vi "SiPM_Data_Analysis.vi"() -> ()   [LabVIEW 2019]
uses:
  <vilib>/Utility/error.llb/DialogType.ctl
  SiPM_Tests_Global_Var.vi
  Data_Analysis_subvis/ESA_Data_Analysis_Global_VIs.vi
  <vilib>/Analysis/NI_AALPro.lvlib
panel:
  out "property names":string[](array[string])
  out "property values":variant[](array[variant])
  out "data":waveform(dbl)[](array[waveform])
  out "Indicator":bool
  in  "Close Session":bool
  in  "Spectrum Calculation":bool=TRUE
  in  "Waveform Nb":u16
  in  "NbSamples":i64=100000 caption="Nb of Samples to Analyze" format="%.0p"
  in  "Refresh":bool
  in  "Load file to display":bool
  in  "Detailed":bool
  in  "Listbox":i32[](listbox) caption="Protn-Neutron_Board_v1.tdms"
  in  "Y-Scale":bool
  out "Nb of Selected Events":dbl step=0.001 format="%#_6p"
  out "Total Nb of Recorded Events":dbl step=0.001 format="%#_6p"
  in  "CH4 Trigger Logic":T1(ring)
  in  "CH4 Trigger Thr":dbl=0.003 caption="CH4 Trigger Thr (V)" step=0.001 format="%#_6p"
  in  "CH3 Trigger Logic":T1(ring)
  in  "CH3 Trigger":dbl=0.003 caption="CH3 Trigger Thr (V)" step=0.001 format="%#_6p"
  in  "CH2 Trigger Logic":T1(ring)
  in  "CH2 Trigger Thr":dbl=0.003 caption="CH2 Trigger Thr (V)" step=0.001 format="%#_6p"
  in  "AutoScale 3":bool
  in  "Update Energy":bool
  out "Energy_Spectr":T2(graph) caption="Spectrum"
  in  "Filter \nON?":bool
  in  "Threshold 2":dbl caption="Max_Value (V)" step=0.001 format="%#_6p"
  in  "Threshold":dbl caption="Energy Threshold (V)" step=0.001 format="%#_6p"
  out "SiPM Waveform":waveform(dbl)[](graph)
  out "Table":string[][](table)
  in  "Bin Min (V)":dbl=-0.0042 step=0.001 format="%#_6p"
  in  "Bin Max (V)":dbl=0.03005 step=0.001 format="%#_6p"
  out "Nb of Channels in Group":i32
  out "group names":string[](array[string])
  out "tdms file out":refnum<k34>
  in  "File contents":string[](tree)
  # "NCSR  DEMOKRITOS\nInstitute of Nuclear and Particle Physics\nDetectors Instrumentation Laboratory"
  # "SiPM Data Analysis"
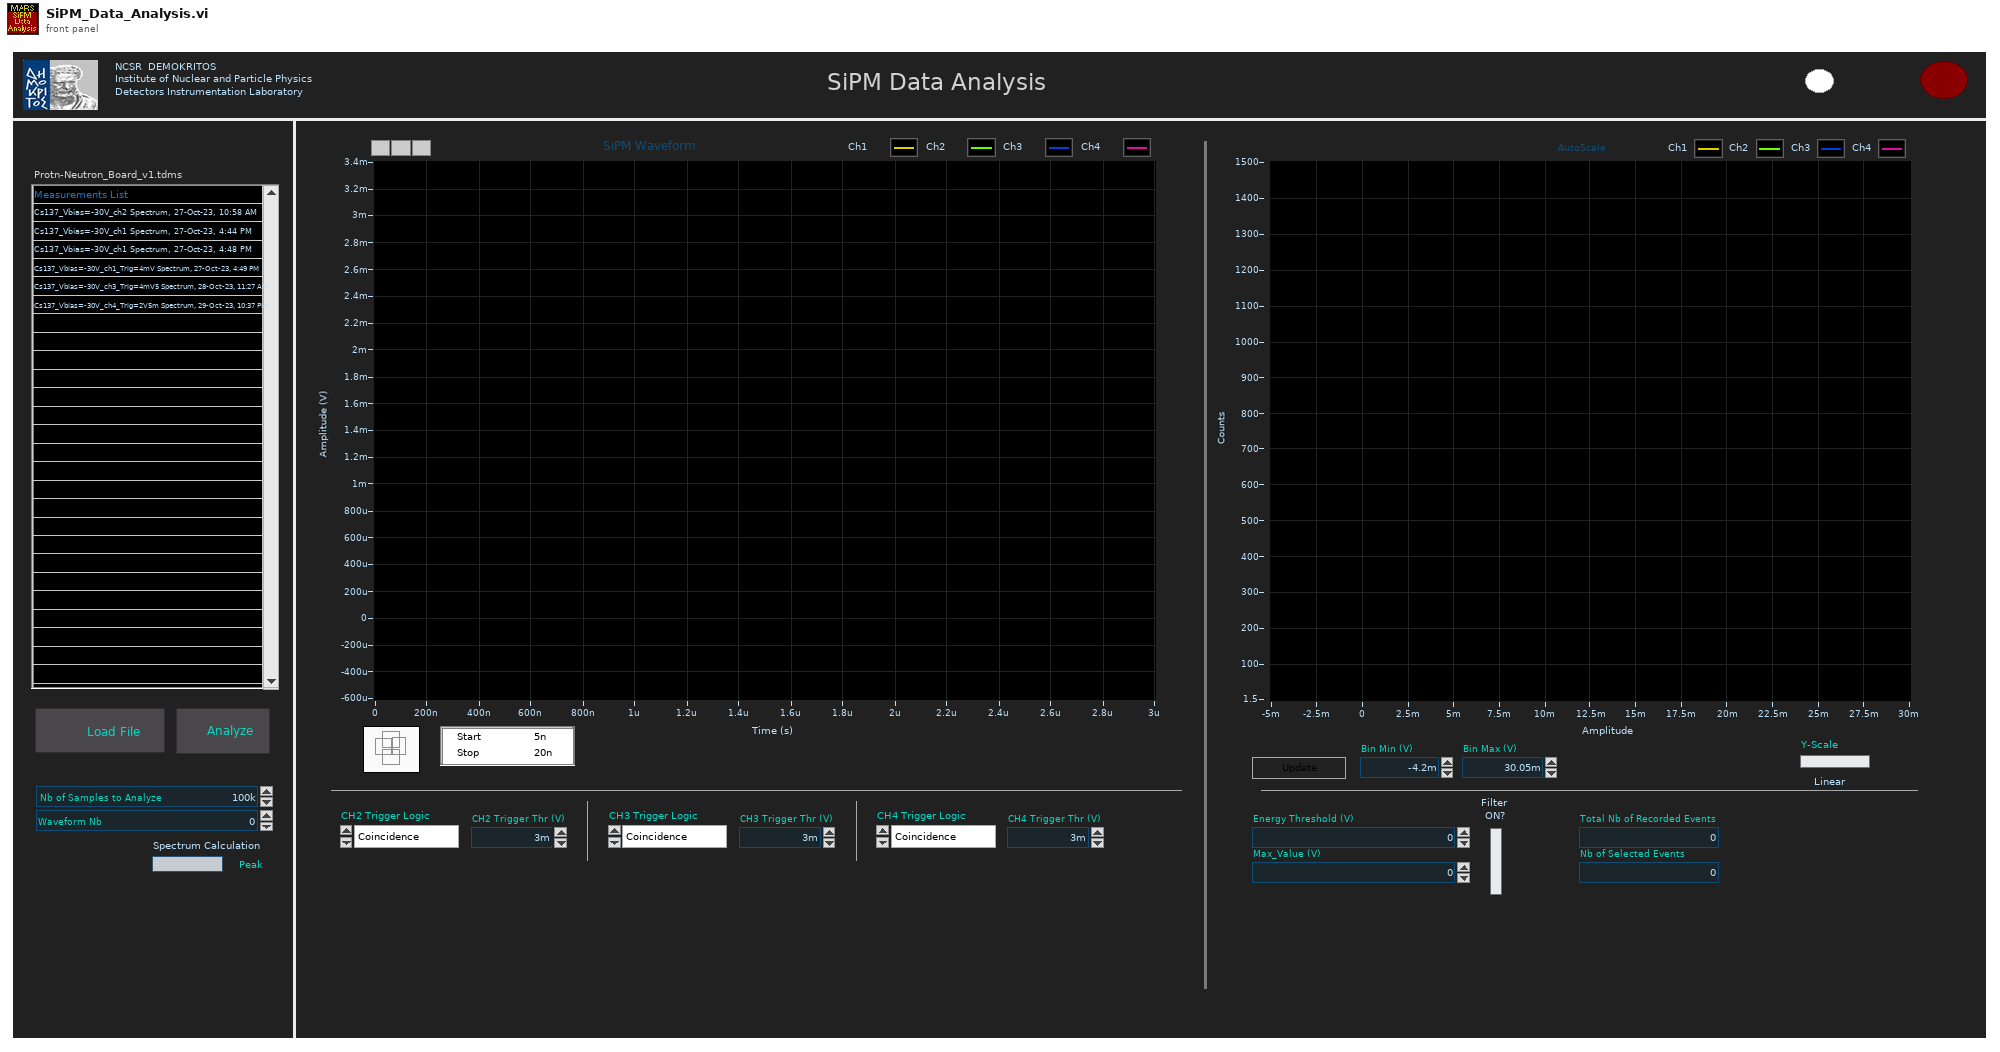
[diagram p1: front panel]
types:
  T1 = enum16{"Coincidence", "Anti-Coincidence", "Don't Care"}
  T2 = cluster{"X Values":dbl[], "Histogram: h(x)":i32[]}[]
  T3 = typedef "DialogType.ctl" = u16
  T4 = enum16{"open", "open or create", "create or replace", "create", "open (read-only)"}
  T5 = cluster{"X Values":dbl[], "Histogram: h(x)":i32[]}
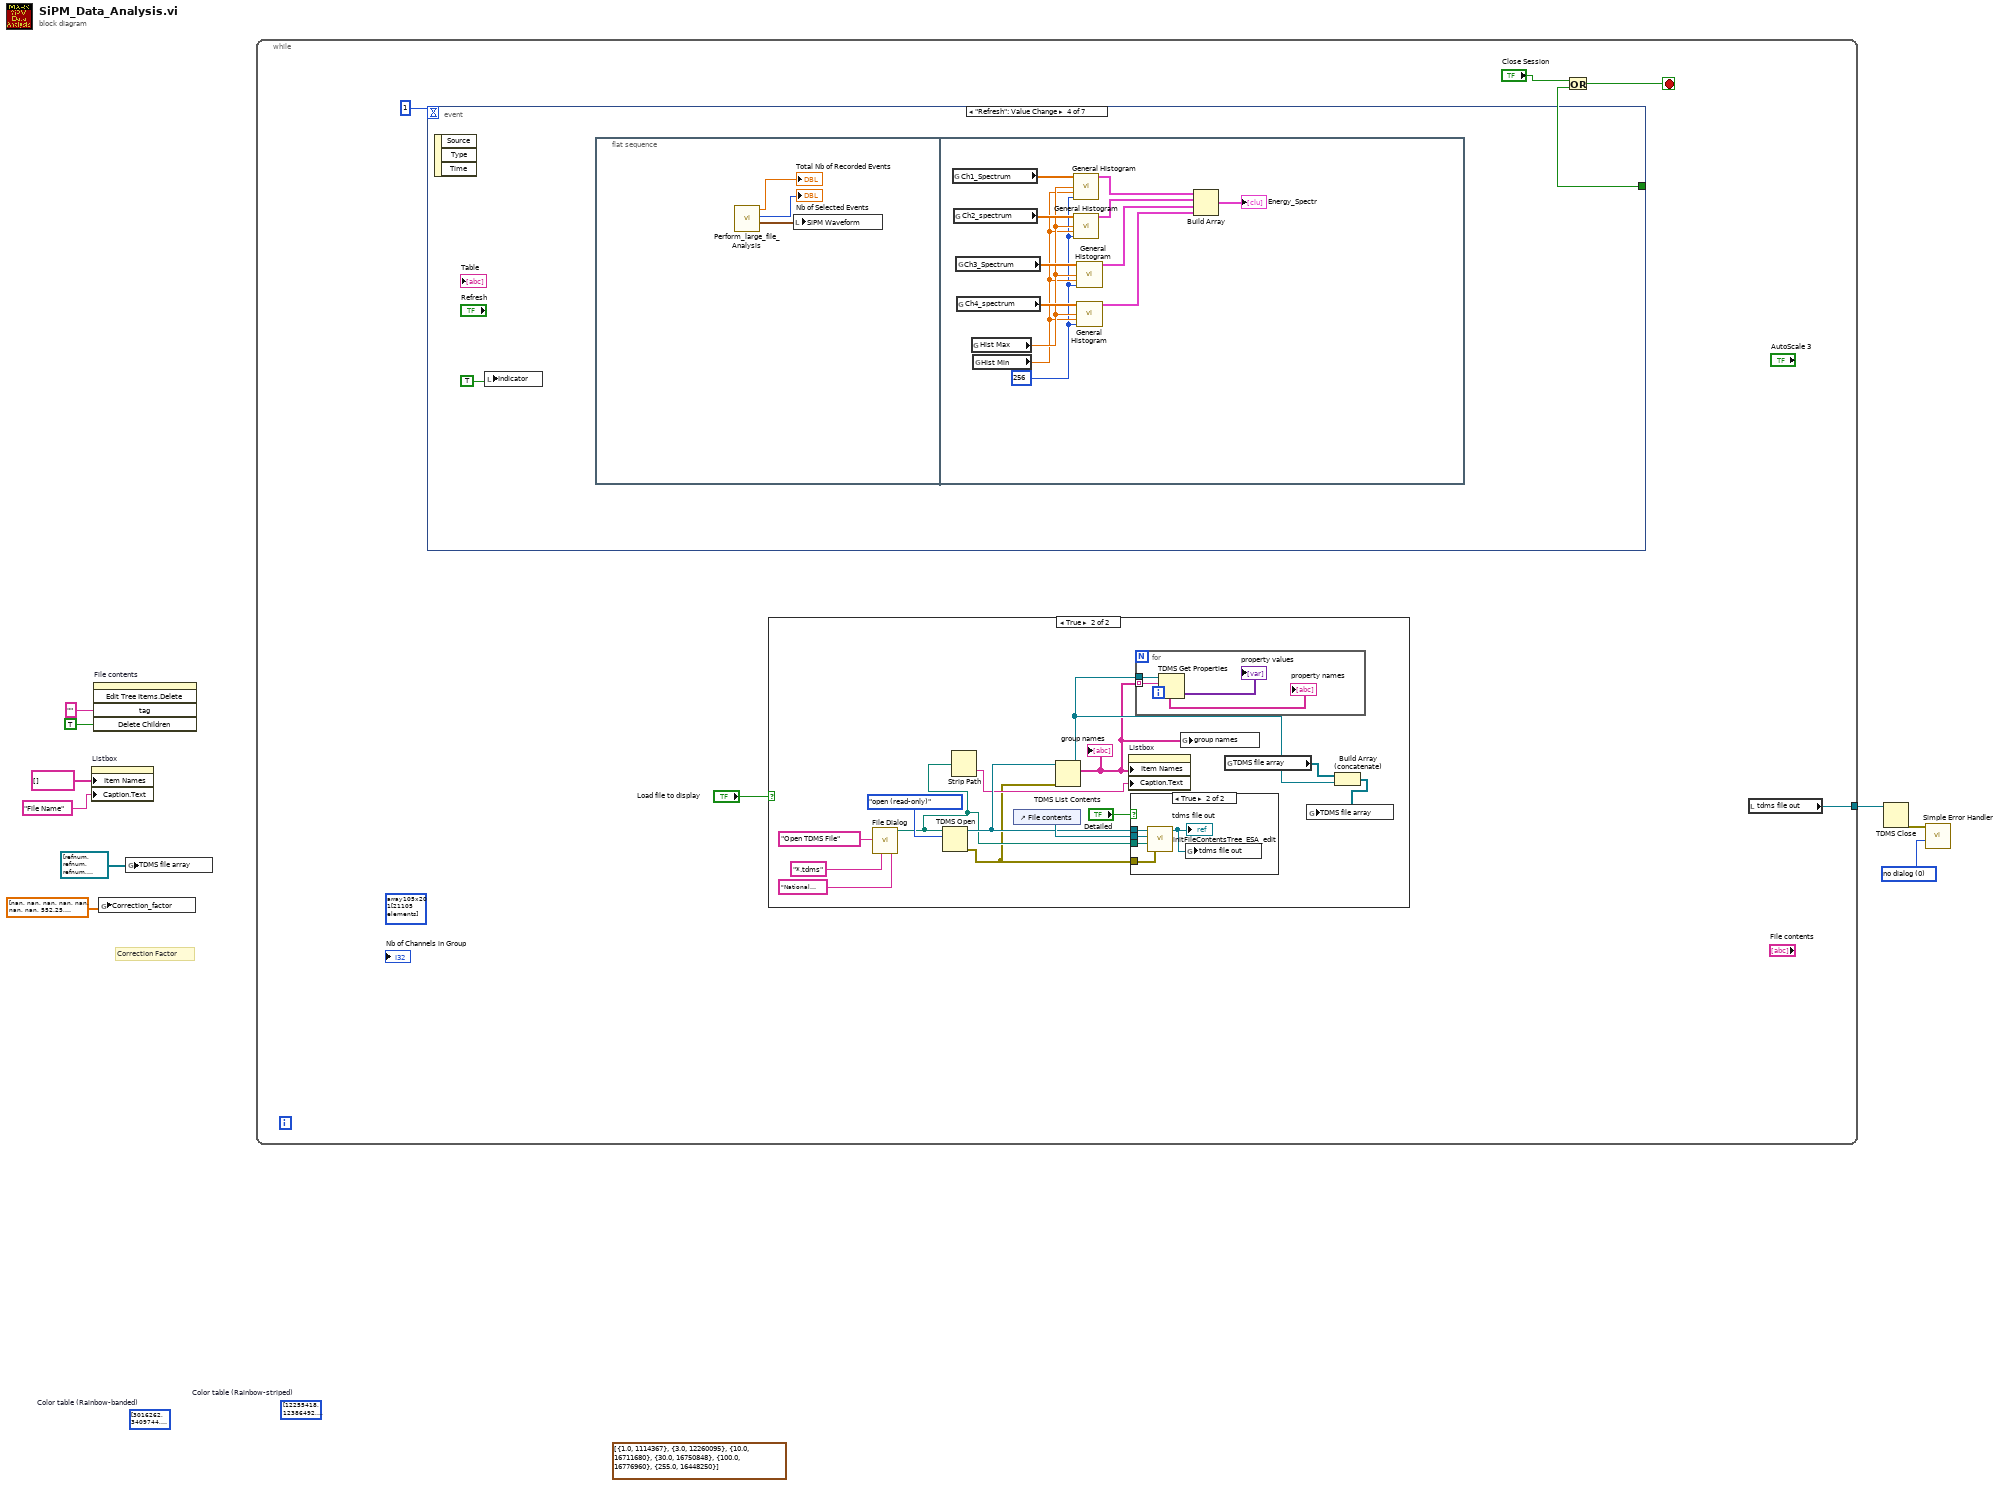
[diagram p0: block diagram]
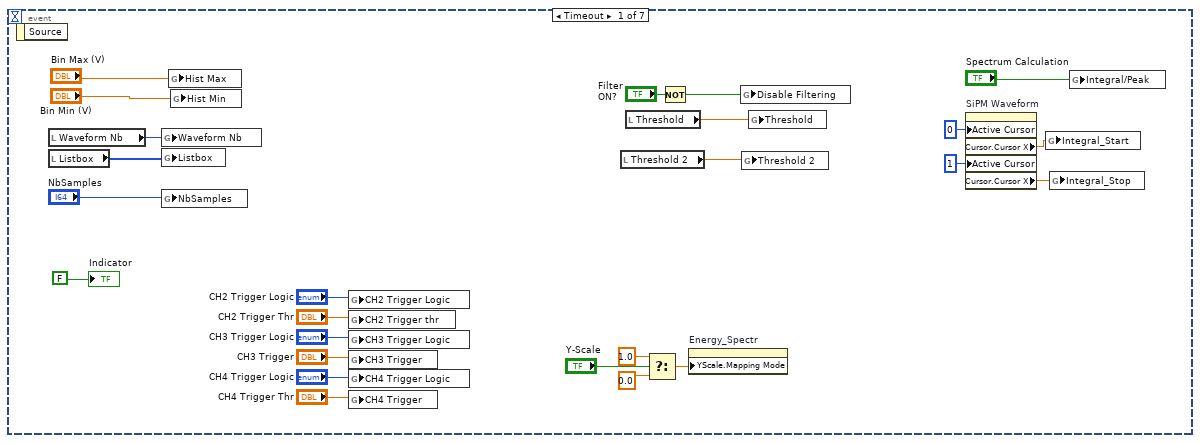
[diagram p2: hidden frame]
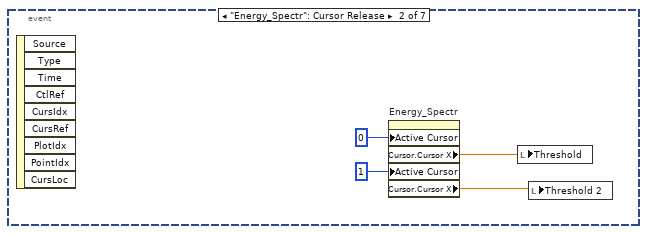
[diagram p3: hidden frame]
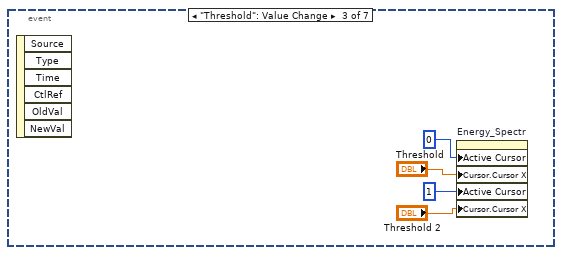
[diagram p4: hidden frame]
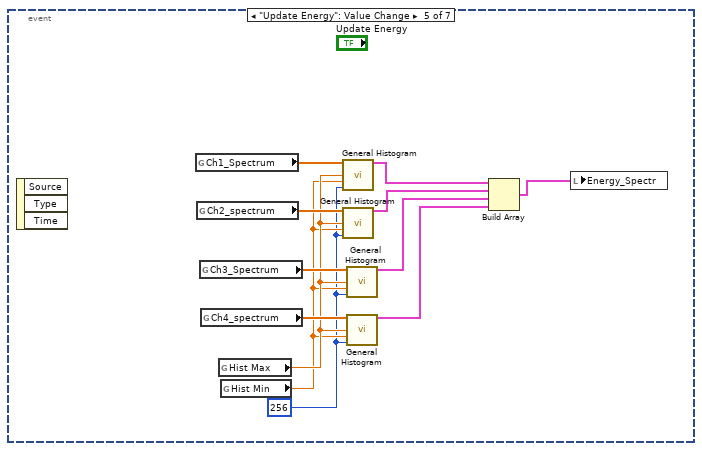
[diagram p5: hidden frame]
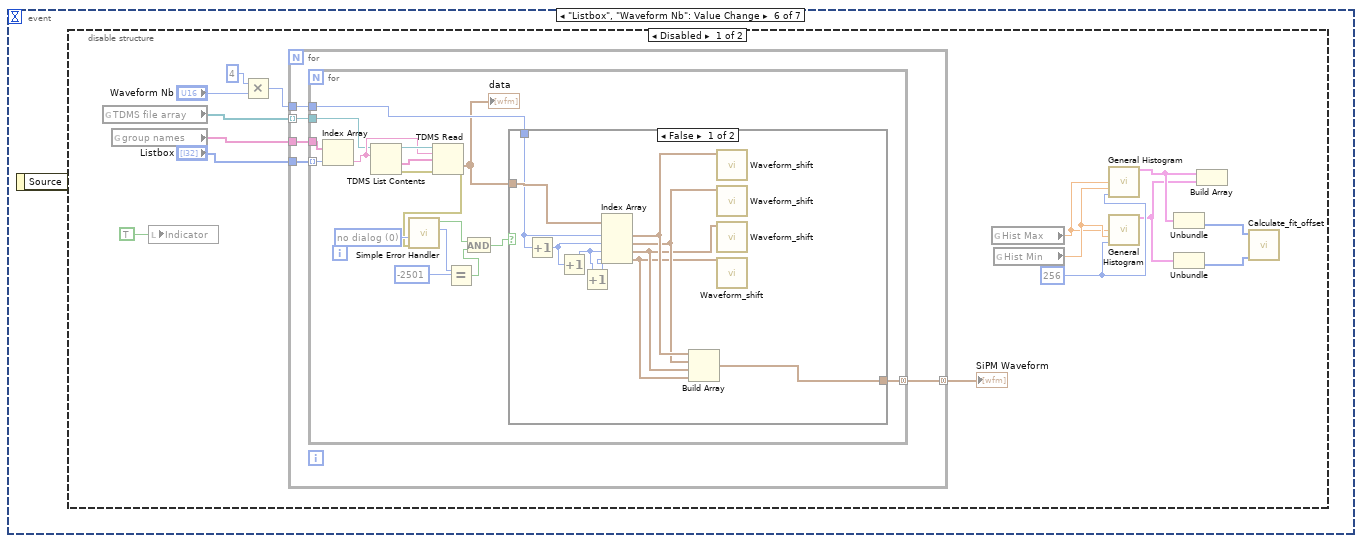
[diagram p6: hidden frame]
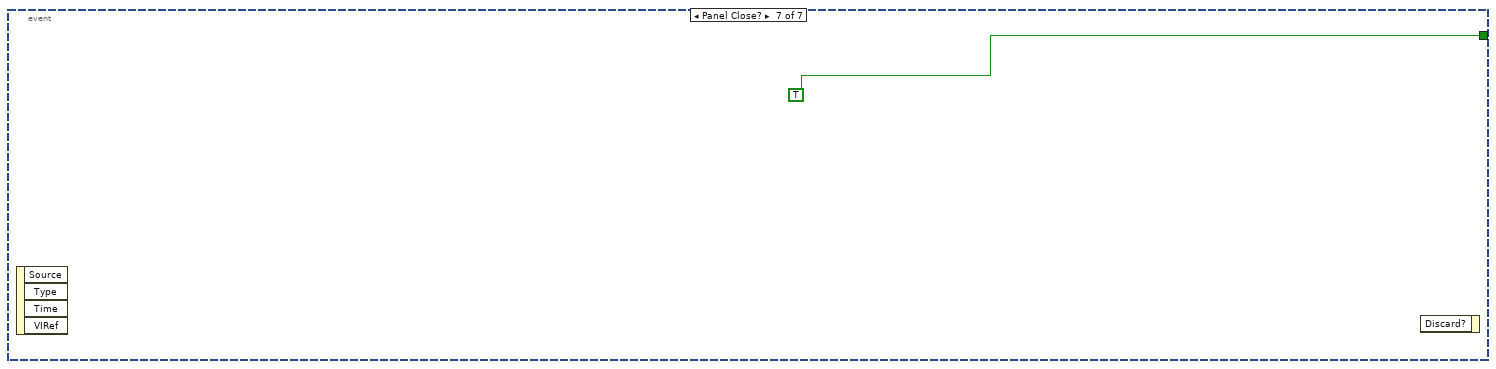
[diagram p9: hidden frame]
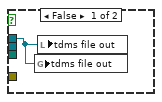
[diagram p11: hidden frame]
diagram:
  w2 = T3 0 items=["no dialog", "OK message", "continue or stop message", "OK message + warnings", "continue/stop + warnings"] ("type of dialog (OK msg:1)")
  (unwired) cluster{dbl, u32}[] [{1.0, 1114367}, {3.0, 12260095}, {10.0, 16711680}, {30.0, 16750848}, {100.0, 16776960}, {255.0, 16448250}] ("Z Scale.Marker Values[]")
  (unwired) u32[] [12255418, 12386492, 12517567, 12320960, 12189888, 12058817, 11927746, 11731139, 11600067, 9175197, 9044125, 11141318, 11010246, 10813639, 10682568, 10551497, 10354890, 10223818, 10092747, 7930019, 7798948, 9633997, 9502926, 9306319, 9175248, 9044176, 8847569, 8716498, 8585427, 6750377, 6619306, 8126677, 7995606, 7798999, 7667927, 7536856, 7340249, 7209178, 7078106, 5505199, 5374128, 6619357, 6488285, 6291678, 6160607, 6029536, 5832929, 5701857, 5570786, 4325557, 4194486, 5112036, 4980965, 4784358, 4653287, 4522215, 4325608, 4194537, 4063466, 3080380, 3014844, 3604716, 3408109, 3277038, 3277038, 3145966, 3014895, 2818288, 2687217, 2556145, 1900738, 1769666, 2097396, 1900789, 1769717, 1638646, 1507575, 1310968, 1179896, 1048825, 721096, 590024, 590075, 393468, 262397, 131326, 255, 1791, 3327, 4863, 5068, 6348, 9471, 11007, 12543, 14079, 15615, 17151, 18687, 20223, 17612, 18636, 25087, 26623, 28159, 29695, 31231, 32767, 34303, 35839, 29900, 31180, 40447, 41983, 43775, 45311, 46847, 48383, 49919, 51455, 42444, 43724, 56063, 57599, 59135, 60671, 62207, 63743, 65535, 65528, 52418, 52413, 65510, 65504, 65498, 65492, 65486, 65480, 65474, 65468, 52369, 52364, 65449, 65443, 65437, 65431, 65425, 65419, 65413, 65407, 52321, 52316, 65389, 65383, 65377, 65371, 65364, 65358, 65352, 65346, 52272, 52267, 65328, 65322, 65316, 65310, 65304, 65298, 65292, 65286, 52224, 314368, 851712, 1244928, 1638144, 2031360, 2424576, 2817792, 3211008, 3604224, 3197952, 3525632, 4783872, 5177088, 5635840, 6029056, 6422272, 6815488, 7208704, 7601920, 6409216, 6736896, 6736896, 8781568, 9174784, 9568000, 9961216, 10354432, 10747648, 11206400, 11599616, 9554944, 9882624, 12779264, 13172480, 13565696, 13958912, 14352128, 14745344, 15138560, 15531776, 12766208, 13093888, 16776960, 16775170, 16773637, 16771847, 16770314, 16768780, 16766991, 16765457, 13411088, 13409810, 16760601, 16758812, 16757278, 16755745, 16753955, 16752422, 16750888, 16749099, 13398052, 13396774, 16744243, 16742704, 16741166, 16739884, 16738345, 16736807, 16735269, 16733730, 13385753, 13384728, 16729371, 16727833, 16726295, 16725012, 16723474, 16721936, 16720397, 16718859, 13373959, 13372677, 16714500, 16712962, 16711680]  # Color table (Rainbow-striped)
  (unwired) u32[] [3016262, 3409744, 4000097, 4721526, 5508493, 6229924, 6820281, 7214025, 7345364, 7279831, 6886611, 6362057, 5640632, 4788132, 4001165, 3214197, 2492769, 2033488, 1640006, 1508930, 1508934, 1640272, 1902945, 2165622, 2428301, 2690980, 2822585, 2888649, 2757844, 2626775, 2299091, 1971145, 1642936, 1249188, 920973, 724086, 592737, 461392, 395846, 396098, 396358, 462928, 595297, 727925, 861069, 994212, 1127608, 1260745, 1328083, 1329111, 1329876, 1264073, 1132217, 999844, 866957, 734070, 600929, 468304, 401734, 401730, 402502, 469584, 603489, 737909, 737909, 872845, 1008036, 1143224, 1277641, 1345747, 1347287, 1347796, 1281225, 1147833, 1013668, 878989, 743798, 609121, 475216, 407878, 407362, 408390, 476496, 611681, 747893, 884877, 1022116, 1158840, 1294793, 1363667, 1365719, 1365202, 1296836, 1161649, 1025178, 888194, 751211, 614742, 479302, 411196, 410168, 411193, 479297, 614732, 750939, 888171, 1025145, 1161350, 1296782, 1364883, 1365906, 1365132, 1296769, 1161588, 1025124, 888147, 751172, 614710, 479276, 411173, 410146, 411170, 479270, 614700, 750900, 888124, 1025091, 1161289, 1296716, 1364813, 1365834, 1365062, 1296703, 1161527, 1025070, 888101, 751133, 614678, 479249, 411149, 410124, 411147, 479244, 614668, 750861, 888078, 1156111, 1488913, 1820947, 2151188, 2414356, 2610196, 2738451, 2668817, 2597903, 2329869, 2061835, 1794313, 1593351, 1459718, 1458694, 1590790, 1921031, 2449673, 3110155, 3902733, 4695055, 5486609, 6211859, 6738708, 7132948, 7197716, 7063827, 6666513, 6136847, 5410061, 4617739, 3957001, 3362823, 2967046, 2900486, 3098118, 3690503, 4546825, 5666059, 6917389, 8233999, 9484305, 10537235, 11326228, 11786004, 11785236, 11785236, 11454739, 10729745, 9675791, 8424717, 7173643, 6054153, 5066759, 4474374, 4342278, 4605190, 5262855, 6380553, 7695883, 9273613, 10785807, 12100625, 13217555, 13874452, 14136340, 13938196, 13214227, 12161553, 10780431, 9267725, 7755531, 6374921, 5257479, 4599814, 4336646, 4599302, 5255943, 6372361, 7685899, 9261837, 10771983, 12085009, 13200659, 13856532, 14118164, 13920276, 13197075, 12145937, 10766351, 9255949, 7745547, 6366729, 5250567, 4593926, 4331014, 4593158, 5249287, 6364169, 7675915, 9249805, 10758159, 12069393, 13183507, 13838612, 14099988, 13902356, 13180179, 12130065, 10752527]  # Color table (Rainbow-banded)
  # "Correction Factor"
  n1 = property on="Listbox" class="LstBox (strict)"("Item Names"=string[] [], "Caption.Text"="File Name") -> ()  [unwired: 2 in, 2 out]
  n2 = invoke on="File contents" class="Tree (strict)" method="Edit Tree Items.Delete"("tag"="" ("Tag"), "Delete Children"=TRUE ("Delete Children?")) -> ()  [unwired: 3 in, 5 out]
  n3 = global write "SiPM_Tests_Global_Var.vi" "Correction_factor"(dbl[] [nan, nan, nan, nan, nan, nan, nan, 552.25, 547.2727272727273, 556.8888888888889, 571.6521739130435, 581.5526315789474, 593.6590909090909, 606.7333333333333, 610.4848484848485, 619.9565217391304, 624.8125, 628.375, 631.8064516129032, 637.0434782608696, 640.92, 643.5, 643.92, 647.7619047619048, 650.1923076923077, 651.5714285714286, 652.375, 654.9130434782609, 656.35, 658.4117647058823, 658.5909090909091, 660.0952380952381, 662.3157894736842, 661.5, 663.4166666666666, 665.8888888888889, 666.0, 666.0, 667.8421052631579, 668.2727272727273, 669.7, 671.4166666666666, 671.2631578947369, 672.2272727272727, 672.0588235294117, 674.0952380952381, 673.0, 674.0526315789474, 675.6111111111111, 677.1578947368421, 677.9411764705883, 676.5263157894736, 677.0666666666667, 678.0, 677.3333333333334, 678.8333333333334, 678.4, 680.0, 680.0666666666667, 680.625, 678.8823529411765, 681.1764705882352, 680.3333333333334, 681.1052631578947, 681.4375, 683.1052631578947, 682.6875, 682.7222222222222, 683.4666666666667, 684.1052631578947, 682.8461538461538, 685.375, 684.5, 684.8333333333334, 683.8, 684.6111111111111, 685.7142857142857, 686.5555555555555, 684.2857142857143, 685.4444444444445, 685.4375, 686.0, 686.375, 687.1176470588235, 685.3125, 685.9333333333333, 687.0, 686.0, 686.1538461538462, 686.75, 686.7272727272727, 686.875, 687.4444444444445, 686.5, 686.3076923076923, 685.8461538461538, 688.3, 688.3571428571429, 685.8571428571429, 688.4166666666666, 687.4, 687.8, 687.1818181818181, 687.9230769230769, 687.5, 688.7857142857143, 685.5714285714286, 686.9090909090909, 688.2, 690.5555555555555, 688.5, 689.6923076923077, 689.6, 690.1111111111111, 692.5, 687.6666666666666, 688.0, 686.0, 690.5, 690.0, 688.6666666666666, nan, 691.75, 682.0, 687.5, 692.5, 690.0, 687.0, 686.3333333333334, 693.5, 689.5, 689.5, nan, nan, 693.0, nan, 686.0, nan, nan, nan, 690.0, 690.0, nan, nan, nan, nan, nan, nan, nan, nan, nan, nan, nan, nan, nan, nan, nan, nan, nan, nan, nan, nan, nan, nan, nan, nan, nan, nan, nan, nan, nan, nan, nan, nan, nan, nan, nan, nan, nan, nan, nan, nan, nan, nan, nan, nan, nan, nan, nan, nan, nan, nan, nan, nan, nan, nan, nan, nan, nan, nan, nan, nan, nan, nan, nan, nan, nan, nan, nan, nan, nan, nan, nan, nan, nan, nan, nan, nan, nan, nan, nan, nan, nan, nan, nan, nan, nan, nan, nan, nan, nan, nan, nan, nan, nan, nan, nan, nan, nan, nan, nan, nan, nan, nan, nan, nan, nan, nan, nan, nan, nan, nan, nan, nan, nan, nan, nan] ("Correction_factor")) -> ()
  n4 = global write "SiPM_Tests_Global_Var.vi" "TDMS file array"(refnum<k34>[] [refnum, refnum, refnum, refnum] ("TDMS file array")) -> ()
  n5 = while {
    tunnel: [w14] -> w9
    stop <- w13 stop-if-true
    (unwired) i32[][] array105x201[21105 elements] ("spectrum")
    n6 = event shown="[3] \"Refresh\": Value Change" {
      selector: _ -> [_ _ _ _ _ _ _]
      dyn-events: _ -> [_ _ _ _ _ _ _]
      timeout: 1 -> [_ _ _ _ _ _ _]
      tunnel: [_ _ _ _ _ _ TRUE ("Stop Button")] -> w12
      event Timeout {
        n7 = event-data() -> ()  [unwired: 1 in, 1 out]
        n8 = local read "Waveform Nb"() -> (w34:u16)
        n9 = local read "Listbox"() -> (w37:i32[])
        n10 = global write "SiPM_Tests_Global_Var.vi" "Waveform Nb"(w34) -> ()
        n11 = global write "ESA_Data_Analysis_Global_VIs.vi" "Listbox"(w37) -> ()
        n12 = global write "SiPM_Tests_Global_Var.vi" "NbSamples"("NbSamples") -> ()
        n13 = global write "SiPM_Tests_Global_Var.vi" "Hist Max"("Bin Max (V)") -> ()
        n14 = global write "SiPM_Tests_Global_Var.vi" "Hist Min"("Bin Min (V)") -> ()
        n15 = global write "SiPM_Tests_Global_Var.vi" "CH2 Trigger Logic"("CH2 Trigger Logic") -> ()
        n16 = global write "SiPM_Tests_Global_Var.vi" "CH2 Trigger thr"("CH2 Trigger Thr") -> ()
        n17 = global write "SiPM_Tests_Global_Var.vi" "CH3 Trigger Logic"("CH3 Trigger Logic") -> ()
        n18 = global write "SiPM_Tests_Global_Var.vi" "CH3 Trigger"("CH3 Trigger") -> ()
        n19 = global write "SiPM_Tests_Global_Var.vi" "CH4 Trigger Logic"("CH4 Trigger Logic") -> ()
        n20 = global write "SiPM_Tests_Global_Var.vi" "CH4 Trigger"("CH4 Trigger Thr") -> ()
        n21 = local read "Threshold 2"() -> (w33:dbl)
        n22 = local read "Threshold"() -> (w35:dbl)
        n23 = Select(t=1.0, s="Y-Scale", f=0.0 ("t")) -> (s? t:f=w19:dbl)
        n24 = Not(x="Filter \nON?") -> (.not. x?=w31:bool)
        n25 = property on="Energy_Spectr" class="XYGraph (strict)"("YScale.Mapping Mode"=w19) -> ()  [unwired: 2 in, 2 out]
        n26 = global write "SiPM_Tests_Global_Var.vi" "Disable Filtering"(w31) -> ()
        n27 = global write "SiPM_Tests_Global_Var.vi" "Threshold 2"(w33) -> ()
        n28 = global write "SiPM_Tests_Global_Var.vi" "Threshold"(w35) -> ()
        n29 = property on="SiPM Waveform" class="WFGraph (strict)"("Active Cursor"=u32 0, "Active Cursor"=u32 1) -> ("Cursor.Cursor X"=w28:dbl, "Cursor.Cursor X"=w27:dbl)  [unwired: 2 in, 2 out]
        n30 = global write "SiPM_Tests_Global_Var.vi" "Integral_Start"(w28) -> ()
        n31 = global write "SiPM_Tests_Global_Var.vi" "Integral_Stop"(w27) -> ()
        n32 = global write "SiPM_Tests_Global_Var.vi" "Integral/Peak"("Spectrum Calculation") -> ()
        "Indicator" <- FALSE ("Indicator")
      }
      event "Energy_Spectr": Cursor Release {
        n33 = event-data() -> ()  [unwired: 1 in, 9 out]
        n34 = property on="Energy_Spectr" class="XYGraph (strict)"("Active Cursor"=u32 0, "Active Cursor"=u32 1) -> ("Cursor.Cursor X"=w44:dbl, "Cursor.Cursor X"=w41:dbl)  [unwired: 2 in, 2 out]
        n35 = local write "Threshold"(w44) -> ()
        n36 = local write "Threshold 2"(w41) -> ()
      }
      event "Threshold": Value Change {
        n37 = event-data() -> ()  [unwired: 1 in, 6 out]
        n38 = property on="Energy_Spectr" class="XYGraph (strict)"("Active Cursor"=u32 0, "Cursor.Cursor X"="Threshold", "Active Cursor"=u32 1, "Cursor.Cursor X"="Threshold 2") -> ()  [unwired: 2 in, 2 out]
      }
      event "Refresh": Value Change {
        n39 = event-data() -> ()  [unwired: 1 in, 3 out]
        n40 = local write "Indicator"(TRUE ("Indicator")) -> ()
        n41 = flat-sequence {
          frame #0 {
            n42 = call "Perform_large_file_Analysis.vi"() -> ("Wvfm"=w52:waveform(dbl)[], "Filtered Nb of Events"=→"Nb of Selected Events":i32, "Total Nb of Events"=→"Total Nb of Recorded Events":dbl)  [unwired: 6 in]
            n43 = local write "SiPM Waveform"(w52) -> ()
          }
          frame #1 {
            w55 = 256 ("# bins")
            n44 = global read "SiPM_Tests_Global_Var.vi" "Ch1_Spectrum"() -> (w63:dbl[])
            n45 = global read "SiPM_Tests_Global_Var.vi" "Ch2_spectrum"() -> (w64:dbl[])
            n46 = global read "SiPM_Tests_Global_Var.vi" "Ch3_Spectrum"() -> (w59:dbl[])
            n47 = global read "SiPM_Tests_Global_Var.vi" "Ch4_spectrum"() -> (w58:dbl[])
            n48 = global read "SiPM_Tests_Global_Var.vi" "Hist Max"() -> (w57:dbl)
            n49 = global read "SiPM_Tests_Global_Var.vi" "Hist Min"() -> (w56:dbl)
            n50 = call <vilib>:"General Histogram.vi"("X"=w63, "max"=w57, "min"=w56, "# bins"=w55) -> ("Histogram Graph"=w61:T5)  [unwired: 7 in, 4 out]
            n51 = call <vilib>:"General Histogram.vi"("X"=w64, "max"=w57, "min"=w56, "# bins"=w55) -> ("Histogram Graph"=w60:T5)  [unwired: 7 in, 4 out]
            n52 = call <vilib>:"General Histogram.vi"("X"=w59, "max"=w57, "min"=w56, "# bins"=w55) -> ("Histogram Graph"=w54:T5)  [unwired: 7 in, 4 out]
            n53 = call <vilib>:"General Histogram.vi"("X"=w58, "max"=w57, "min"=w56, "# bins"=w55) -> ("Histogram Graph"=w53:T5)  [unwired: 7 in, 4 out]
            n54 = Build Array(w61, w60, w54, w53) -> (→"Energy_Spectr":T2)
          }
        }
      }
      event "Update Energy": Value Change {
        w68 = 256 ("# bins")
        n55 = event-data() -> ()  [unwired: 1 in, 3 out]
        n56 = global read "SiPM_Tests_Global_Var.vi" "Ch1_Spectrum"() -> (w75:dbl[])
        n57 = global read "SiPM_Tests_Global_Var.vi" "Ch2_spectrum"() -> (w76:dbl[])
        n58 = global read "SiPM_Tests_Global_Var.vi" "Ch3_Spectrum"() -> (w72:dbl[])
        n59 = global read "SiPM_Tests_Global_Var.vi" "Ch4_spectrum"() -> (w71:dbl[])
        n60 = global read "SiPM_Tests_Global_Var.vi" "Hist Max"() -> (w70:dbl)
        n61 = global read "SiPM_Tests_Global_Var.vi" "Hist Min"() -> (w69:dbl)
        n62 = call <vilib>:"General Histogram.vi"("X"=w75, "max"=w70, "min"=w69, "# bins"=w68) -> ("Histogram Graph"=w74:T5)  [unwired: 7 in, 4 out]
        n63 = call <vilib>:"General Histogram.vi"("X"=w76, "max"=w70, "min"=w69, "# bins"=w68) -> ("Histogram Graph"=w73:T5)  [unwired: 7 in, 4 out]
        n64 = call <vilib>:"General Histogram.vi"("X"=w72, "max"=w70, "min"=w69, "# bins"=w68) -> ("Histogram Graph"=w67:T5)  [unwired: 7 in, 4 out]
        n65 = call <vilib>:"General Histogram.vi"("X"=w71, "max"=w70, "min"=w69, "# bins"=w68) -> ("Histogram Graph"=w66:T5)  [unwired: 7 in, 4 out]
        n66 = Build Array(w74, w73, w67, w66) -> (w65:T2)
        n67 = local write "Energy_Spectr"(w65) -> ()
      }
      event "Listbox", "Waveform Nb": Value Change {
        n68 = event-data() -> ()  [unwired: 1 in, 1 out]
        n69 = disable-structure shown="Disabled" {
          frame Disabled {
            w81 = 256 ("# bins")
            n70 = global read "SiPM_Tests_Global_Var.vi" "TDMS file array"() -> (w90:refnum<k34>[])
            n71 = global read "ESA_Data_Analysis_Global_VIs.vi" "group names"() -> (w91:string[])
            n72 = local write "Indicator"(TRUE ("Indicator")) -> ()
            n73 = Multiply(x=4, y="Waveform Nb") -> (x*y=w86:i32)
            n74 = for {
              tunnel: "Listbox" -> [w96]
              tunnel: w91 -> [w95]
              tunnel: w90 -> [w94] mode=indexing
              tunnel: [w93] -> w84 mode=concatenating
              tunnel: w86 -> [w92]
              n75 = for {
                tunnel: w96 -> [w109] mode=indexing
                tunnel: w95 -> [w108]
                tunnel: w94 -> [w107]
                tunnel: [w106] -> w93 mode=concatenating
                tunnel: w92 -> [w98]
                w105 = T3 0 items=["no dialog", "OK message", "continue or stop message", "OK message + warnings", "continue/stop + warnings"] ("type of dialog (OK msg:1)")
                n76 = Index Array(array=w108, index=w109) -> (element=w112:string)
                n77 = TDMS List Contents(6:w112, 7:w107) -> (0:w110:errorcluster, 1:w111:string[], 3:w113:refnum<k34>)  [unwired: 1 in, 1 out]
                n78 = TDMS Read(0:w113, 5:w112, 7:w111, 11:w110) -> (10:w97:waveform(dbl)[], 15:w101:errorcluster)  [unwired: 4 in, 4 out]
                "data" <- w97
                n79 = call <vilib>:"Simple Error Handler.vi"("type of dialog (OK msg:1)"=w105, "error in (no error)"=w101) -> ("error?"=w100:bool, "code out"=w104:i32)  [unwired: 3 in, 3 out]
                n80 = Equal?(x=w104, y=-2501) -> (x = y?=w102:bool)
                n81 = And(x=w100, y=w102) -> (x .and. y?=w99:bool)
                n82 = case shown="False" w99 {
                  tunnel: w97 -> [w123 _]
                  tunnel: [w119 _] -> w106
                  tunnel: w98 -> [w122 _]
                  frame False {
                    n83 = Increment(x=w122) -> (x+1=w118:i32)
                    n84 = Increment(x=w118) -> (x+1=w116:i32)
                    n85 = Increment(x=w116) -> (x+1=w117:i32)
                    n86 = Index Array(array=w123, index #1=w122, index #2=w118, index #3=w116, index #4=w117) -> (element #1=w121:waveform(dbl), element #2=w120:waveform(dbl), element #3=w115:waveform(dbl), element #4=w114:waveform(dbl))
                    n87 = Build Array(w121, w120, w115, w114) -> (w119:waveform(dbl)[])
                    n88 = call "Waveform_shift.vi"("Waveform_in"=w121) -> ()  [unwired: 9 in, 1 out]
                    n89 = call "Waveform_shift.vi"("Waveform_in"=w120) -> ()  [unwired: 9 in, 1 out]
                    n90 = call "Waveform_shift.vi"("Waveform_in"=w115) -> ()  [unwired: 9 in, 1 out]
                    n91 = call "Waveform_shift.vi"("Waveform_in"=w114) -> ()  [unwired: 9 in, 1 out]
                  }
                  frame True {
                  }
                }
              }
            }
            "SiPM Waveform" <- w84
            n92 = global read "SiPM_Tests_Global_Var.vi" "Hist Max"() -> (w82:dbl)
            n93 = global read "SiPM_Tests_Global_Var.vi" "Hist Min"() -> (w83:dbl)
            n94 = call <vilib>:"General Histogram.vi"("max"=w82, "min"=w83, "# bins"=w81) -> ("Histogram Graph"=w80:T5)  [unwired: 8 in, 4 out]
            n95 = call <vilib>:"General Histogram.vi"("max"=w82, "min"=w83, "# bins"=w81) -> ("Histogram Graph"=w79:T5)  [unwired: 8 in, 4 out]
            n96 = Unbundle(w80) -> ("Histogram: h(x)"=w78:i32[])  [unwired: 1 out]
            n97 = Unbundle(w79) -> ("Histogram: h(x)"=w77:i32[])  [unwired: 1 out]
            n98 = Build Array(w80, w79) -> ()  [unwired: 1 out]
            n99 = call "Calculate_fit_offset.vi"("baseline1"=w78, "baseline2"=w77) -> ()  [unwired: 4 in, 4 out]
          }
          frame Enabled {
          }
        }
      }
      event Panel Close? {
        n100 = event-data() -> ()  [unwired: 1 in, 4 out]
        n101 = event-data() -> ()  [unwired: 2 in, 1 out]
      }
    }
    n102 = case shown="True" "Load file to display" {
      frame False {
      }
      frame True {
        n103 = call "File Dialog"("prompt"="Open TDMS File" ("prompt tdms"), "pattern (all files)"="*.tdms", "pattern label"="National Instruments TDM Streaming" ("pattern label tdms")) -> ("selected path"=w132:path)  [unwired: 4 in, 8 out]
        n104 = TDMS Open(10:T4."open (read-only)" ("operation (0:open)"), 11:w132) -> (0:w129:errorcluster, 3:w133:refnum<k34>)  [unwired: 5 in]
        n105 = Strip Path(path=w132) -> (name=w131:string)  [unwired: 1 out]
        n106 = control-ref of="File contents"() -> (w138:refnum<vi>)
        n107 = TDMS List Contents(4:w129, 7:w133) -> (2:w125:string[], 3:w126:refnum<k34>)  [unwired: 1 in, 2 out]
        "group names" <- w125
        n108 = property on="Listbox" class="LstBox (strict)"("Item Names"=w125, "Caption.Text"=w131) -> ()  [unwired: 2 in, 2 out]
        n109 = case shown="True" "Detailed" {
          tunnel: w138 -> [_ w148]
          tunnel: w129 -> [_ w147]
          tunnel: w132 -> [_ w146]
          tunnel: w133 -> [w143 w145]
          frame False {
            n110 = global write "ESA_Data_Analysis_Global_VIs.vi" "tdms file out"(w143) -> ()
            n111 = local write "tdms file out"(w143) -> ()
          }
          frame True {
            n112 = call "initFileContentsTree_ESA_edit.vi"("error in (no error)"=w147, "file path"=w146, "Tree Refnum"=w148, "tdms file"=w145) -> ("tdms file out"=w144:refnum<k34>)  [unwired: 2 in, 1 out]
            "tdms file out" <- w144
            n113 = global write "ESA_Data_Analysis_Global_VIs.vi" "tdms file out"(w144) -> ()
          }
        }
        n114 = for {
          tunnel: w126 -> [w142]
          tunnel: w125 -> [w139] mode=indexing
          n115 = TDMS Get Properties(10:w139, 11:w142) -> (4:→"property values":variant[], 6:→"property names":string[])  [unwired: 4 in, 4 out]
        }
        n116 = global write "ESA_Data_Analysis_Global_VIs.vi" "group names"(w125) -> ()
        n117 = global read "SiPM_Tests_Global_Var.vi" "TDMS file array"() -> (w128:refnum<k34>[])
        n118 = Build Array (concatenate)(w128, w126) -> (w127:refnum<k34>[])
        n119 = global write "SiPM_Tests_Global_Var.vi" "TDMS file array"(w127) -> ()
      }
    }
    n120 = Or(x="Close Session", y=w12) -> (x .or. y?=w13:bool)
    n121 = local read "tdms file out"() -> (w14:refnum<k34>)
  }
  n122 = TDMS Close(11:w9) -> (0:w3:errorcluster)  [unwired: 1 in, 1 out]
  n123 = call <vilib>:"Simple Error Handler.vi"("type of dialog (OK msg:1)"=w2, "error in (no error)"=w3) -> ()  [unwired: 3 in, 5 out]
